vi "RTS Read Base File.vi"(8 "Error In":errorcluster, 11 "File Location":path) -> (0 "Error Out":errorcluster, 3 "all rows":dbl[][](array[numeric]))   [LabVIEW 2016]
uses:
  <vilib>/Utility/file.llb/Read Delimited Spreadsheet (DBL).vi
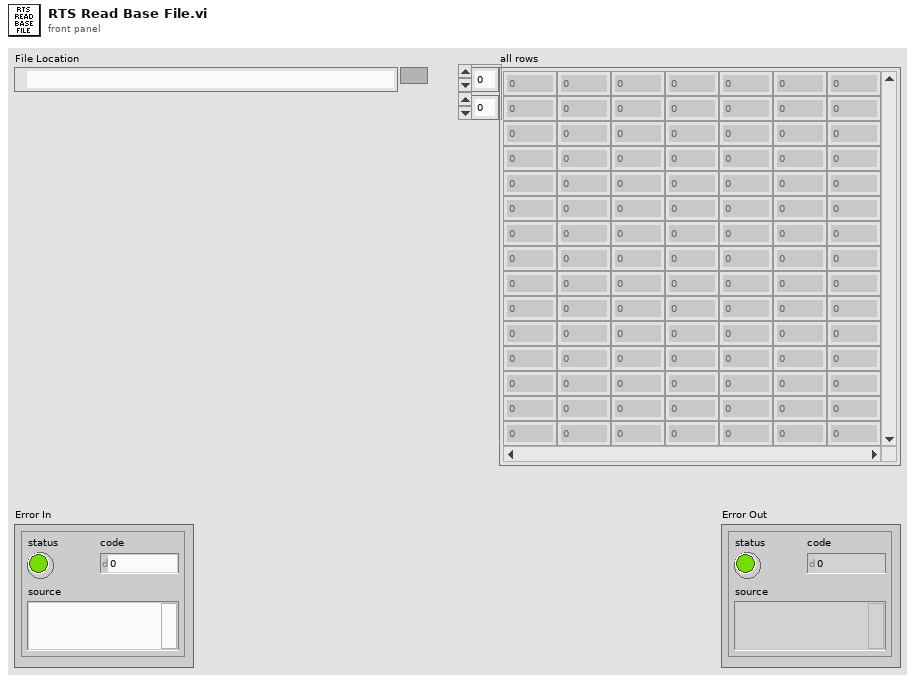
[diagram p1: front panel]
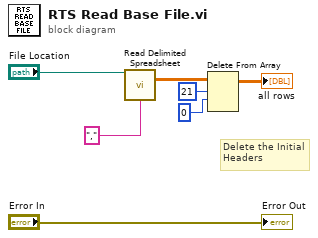
[diagram p0: block diagram]
diagram:
  # "Delete the Initial\nHeaders"
  n1 = call-poly <vilib>:"Read Delimited Spreadsheet.vi"("file path (dialog if empty)"="File Location", "delimiter (\\t)"="," ("delimiter (\\t)")) -> ("all rows"=w4:dbl[][])  [unwired: 8 in, 5 out]
  n2 = Delete From Array(array=w4, length=21, index (row)=0 ("disabled index (col)")) -> (array with subset deleted=→"all rows":dbl[][])  [unwired: 1 in, 1 out]
  "Error Out" <- "Error In"
